vi "Add.vi"(10 "y":dbl, 11 "x":dbl) -> (2 "x+y":dbl)   [LabVIEW 2019]
panel:
  out "x .and. y?":bool
  in  "Cluster":cluster{"Numeric Control":dbl, "Boolean":bool}
  # "eva = best anime"
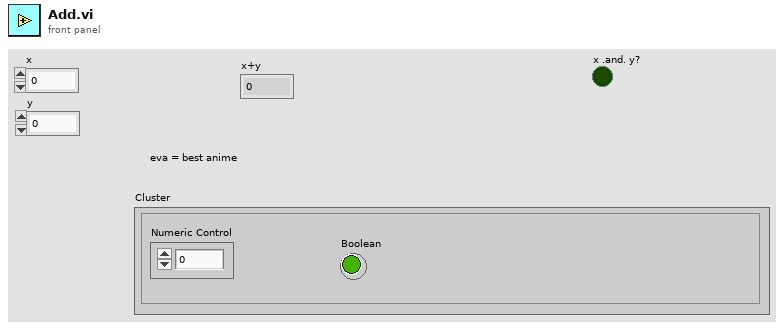
[diagram p1: front panel]
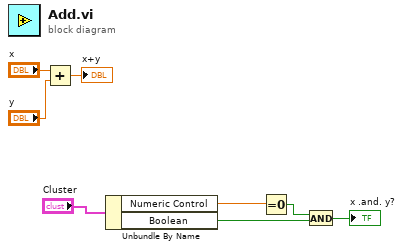
[diagram p0: block diagram]
diagram:
  n1 = Add(x="x", y="y") -> (x+y=→"x+y":dbl)
  n2 = Unbundle By Name("Cluster") -> ("Numeric Control"=w4:dbl, "Boolean"=w3:bool)
  n3 = Equal To 0?(x=w4) -> (x = 0?=w2:bool)
  n4 = And(x=w2, y=w3) -> (x .and. y?=→"x .and. y?":bool)
